vi "macro_TrajectoryConstraint_CentripAccel.vi"   [LabVIEW 2019, in "Trajectory_Library.lvlib"]
uses:
  Trajectory_Library.lvlib
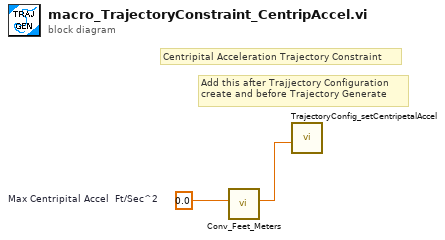
[diagram p0: block diagram]
diagram:
  w2 = 0.0  # Max Centripital Accel  Ft/Sec^2
  # "Centripital Acceleration Trajectory Constraint"
  # "Add this after Trajjectory Configuration\ncreate and before Trajectory Generate"
  n1 = call "Conv_Feet_Meters.vi"("Feet"=w2) -> ("Meters"=w1:dbl)  [unwired: 10 in]
  n2 = call "TrajectoryConfig_setCentripetalAccel.vi"("Max Cent Accel"=w1) -> ()  [unwired: 10 in, 1 out]
